vi "LCB Set Device Property.vi"(7 "Property ID":i32, 8 "error in (no error)":errorcluster caption="Fehler (Eingang, kein Fehler)", 10 "Value":dbl, 11 "Device Handle":i64) -> (0 "error out":errorcluster caption="Fehler (Ausgang)", 3 "Device Handle Out":i64)   [LabVIEW 2021, in "labbCAN_Bus_API.lvlib"]
doc: "LCB_Func long __stdcall LCB_SetCommState(dev_hdl hDev_in,\n unsigned char CommState);"
uses:
  labbCAN_Bus_API.lvlib
  labbCAN_Bus_API.dll
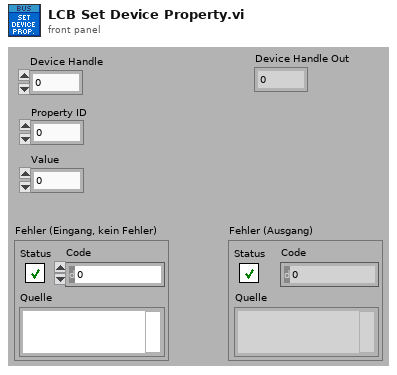
[diagram p1: front panel]
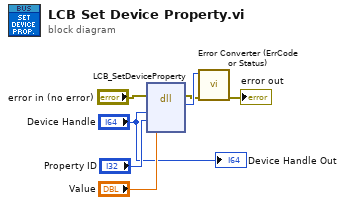
[diagram p0: block diagram]
diagram:
  n1 = dll-call lib="C:/Users/olaja/AppData/Local/CETONI_SDK/labbCAN_Bus_API.*" fn="LCB_SetDeviceProperty"(error in="error in (no error)", "DeviceHandle"="Device Handle", "PropertyId"="Property ID", "Value"="Value") -> (error out=w5:errorcluster, "Rückgabetyp"=w6:i32)  [unwired: 5 in, 1 out]
  n2 = call "Error Converter (ErrCode or Status).vi"("error in (no error)"=w5, "error code"=w6) -> ("error out"=→"error out":errorcluster)  [unwired: 9 in]
  "Device Handle Out" <- "Device Handle"
